vi "JUnit Simple.vi"() -> ()   [LabVIEW 2013]
doc: "This example provides a simple example for <B>JUnit XML</B>."
uses:
  JUnit XML/Test Suite/Test Suite.lvclass
  <vilib>/xml/Close Reference(Node).vi
  <vilib>/xml/NI_XML.lvlib
  JUnit XML/Test Case/Test Case.lvclass
  <resource>/objmgr/DOMUserDefRef.rc
panel:
  out "XML":string
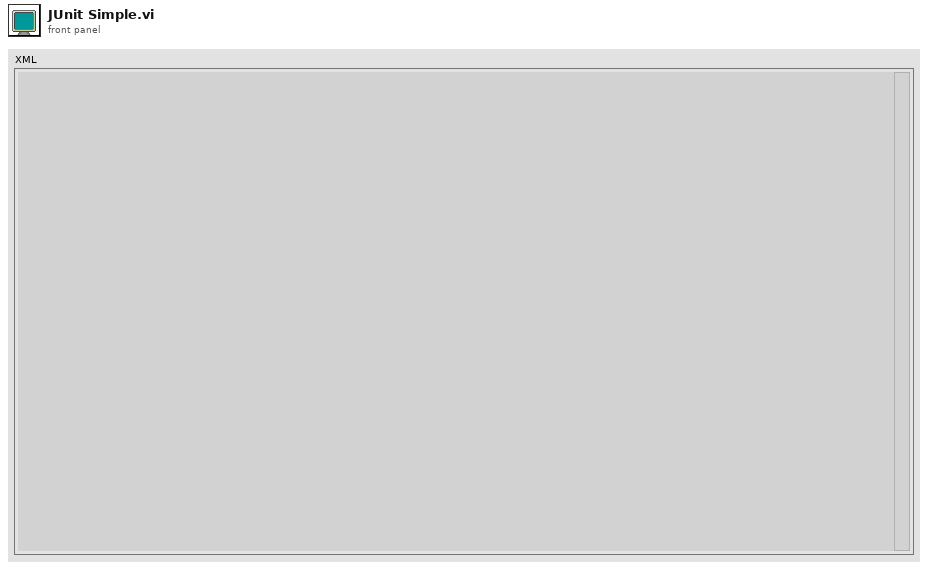
[diagram p1: front panel]
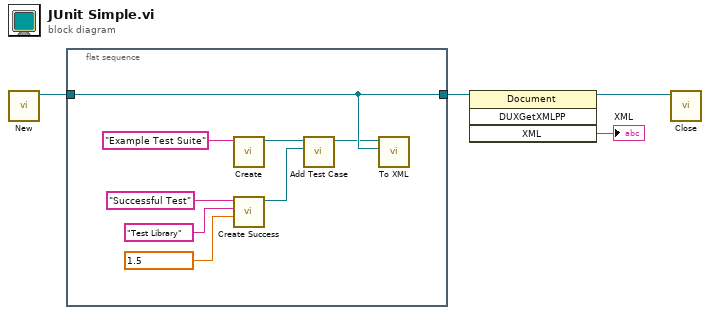
[diagram p0: block diagram]
diagram:
  n1 = call <vilib>:"New.vi"() -> ("DOM document out"=w4:refnum<k20>)  [unwired: 8 in, 1 out]
  n2 = flat-sequence {
    tunnel: w4 -> [w6]
    tunnel: [w6] -> w2
    frame #0 {
      n3 = call "Create.vi"("Name"="Example Test Suite") -> ("Test Suite"=w8:refnum<class "Test Suite.lvclass">)  [unwired: 9 in, 1 out]
      n4 = call "Create Success.vi"("Time"=1.5, "Classname"="Test Library", "Name"="Successful Test") -> ("Test Case"=w7:refnum<class "Test Case.lvclass">)  [unwired: 7 in, 1 out]
      n5 = call "Add Test Case.vi"("Test Case"=w7, "Test Suite in"=w8) -> ("Test Suite out"=w5:refnum<class "Test Suite.lvclass">)  [unwired: 8 in, 1 out]
      n6 = call-dynamic "To XML.vi"("Parent"=w6, "Test Suite in"=w5) -> ()  [unwired: 9 in, 1 out]
    }
  }
  n7 = invoke class="Document" method="DUXGetXMLPP"(reference=w2) -> (reference out=w3:refnum<k20>, "XML"=→"XML":string)  [unwired: 3 in, 2 out]
  n8 = call-poly <vilib>:"Close.vi"("node"=w3) -> ()  [unwired: 8 in, 1 out]
